vi "Get_Triple_Delays.vi"(4 "Delay Second-Third":dbl, 5 "Delays012 in":dbl[](array[numeric]), 6 "Third TimeTag":dbl, 7 "First Timetag":dbl, 9 "C012 in":u32, 10 "Coincidence Window":dbl, 11 "Second TimeTag":dbl) -> (2 "C012 out":u32, 3 "Delays012 out":dbl[](array[numeric]))   [LabVIEW 2023]
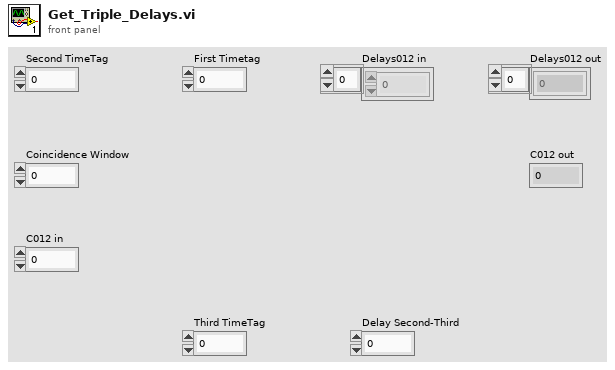
[diagram p1: front panel]
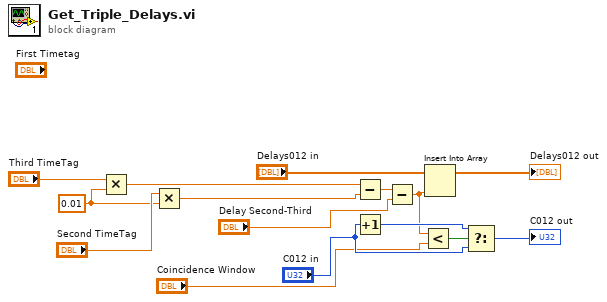
[diagram p0: block diagram]
diagram:
  w5 = 0.01 ("y")
  n1 = Multiply(x="Third TimeTag", y=w5) -> (x*y=w8:dbl)
  n2 = Multiply(x="Second TimeTag", y=w5) -> (x*y=w6:dbl)
  n3 = Subtract(x=w8, y=w6) -> (x-y=w4:dbl)
  n4 = Increment(x="C012 in") -> (x+1=w2:u32)
  n5 = Subtract(x=w4, y="Delay Second-Third") -> (x-y=w1:dbl)
  n6 = Less?(x=w1, y="Coincidence Window") -> (x < y?=w3:bool)
  n7 = Insert Into Array(array="Delays012 in", new element=w1) -> (→"Delays012 out":dbl[])  [unwired: 1 in]
  n8 = Select(t=w2, s=w3, f="C012 in") -> (s? t:f=→"C012 out":u32)
